vi "Manipulator Immediate.vi"(7 "Description":string, 8 "Command Info In":T1, 9 "Feedwheel":dbl, 10 "Flywheel":dbl, 11 "Intake":dbl) -> (0 "Command Info Out":T1)   [LabVIEW 2018]
doc: "This template is useful for immediate subsystem actions that do not need deadband filtering\n\nBe sure to right-click and select New from Template and save with a new command name."
uses:
  <vilib>/Rock Robotics/WPI/Framework/Command Status Info.ctl
  <vilib>/Rock Robotics/WPI/Framework/Completion Status.ctl
  <vilib>/Rock Robotics/WPI/Framework/Completion Notifier.ctl
  MountainGoatProtoCode/Manipulator/Implementation/Manipulator Setpoints.ctl
  Implementation/Manipulator Operations.ctl
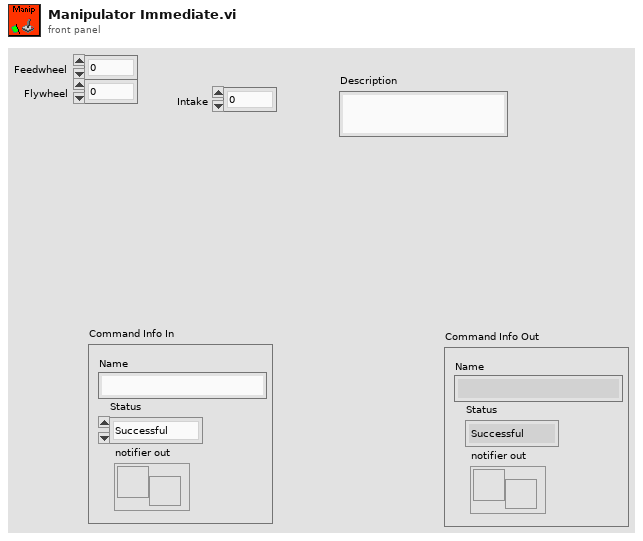
[diagram p1: front panel]
types:
  T1 = typedef "Command Status Info.ctl" = cluster{"Name":string, "Status":T2, "notifier out":T3}
  T2 = typedef "Completion Status.ctl" = enum16{"Successful", "Aborted", "Incomplete"}
  T3 = typedef "Completion Notifier.ctl" = refnum<notifier>
  T4 = typedef "Manipulator Setpoints.ctl" = cluster{"Operation":T5, "Intake":dbl, "Feedwheel":dbl, "Flywheel":dbl, "Duration":dbl}
  T5 = typedef "Manipulator Operations.ctl" = enum16{"Reserve", "Read Current", "Immediate"}
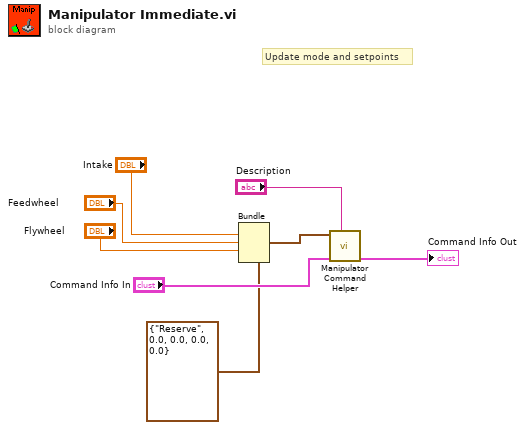
[diagram p0: block diagram]
diagram:
  # "Update mode and setpoints"
  n1 = Bundle(cluster=T4 {"Operation"=enum."Reserve", "Intake"=0.0, "Feedwheel"=0.0, "Flywheel"=0.0, "Duration"=0.0} ("SubSystem Data"), "Intake"="Intake", "Feedwheel"="Feedwheel", "Flywheel"="Flywheel") -> (w3:T4)  [unwired: 2 in]
  n2 = call "Manipulator Command Helper.vi"("Description"="Description", "Command Info In"="Command Info In", "SubSystem Data"=w3) -> ("Command Info Out"=→"Command Info Out":T1)  [unwired: 6 in, 2 out]
